vi "test Deploy Scripted System Definition.vi"(8 "error in (no error)":errorcluster, 11 "TestCase in":refnum<class "Switch Scripting System Tests.lvclass">=refnum) -> (0 "error out":errorcluster, 3 "TestCase out":refnum<class "Switch Scripting System Tests.lvclass">)   [LabVIEW 2017, in "Switch Scripting.lvlib" / "Switch Scripting System Tests.lvclass"]
uses:
  Switch Scripting System Tests.lvclass
  Switch Scripting System Tests.lvclass/Switch Scripting System Tests.ctl
  NationalInstruments.VeriStand.SystemDefinitionAPI
  <vilib>/addons/_JKI Toolkits/VI Tester/TestCase.llb/TestCase.lvclass
  C:/Program Files (x86)/National Instruments/LabVIEW 2017/vi.lib/addons/_JKI Toolkits/VI Tester/TestCase.llb/TestCase.lvclass
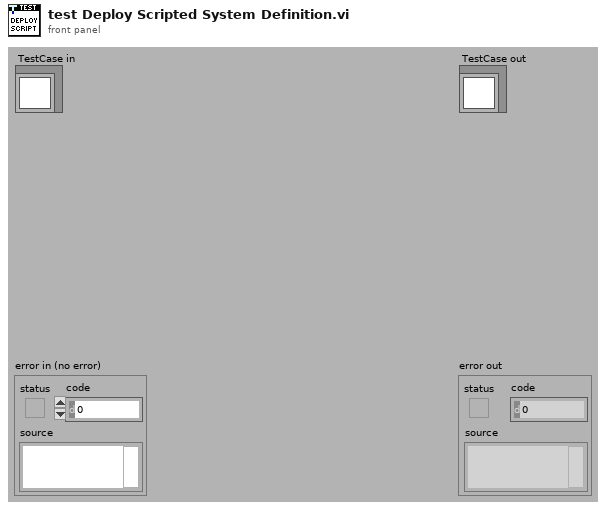
[diagram p1: front panel]
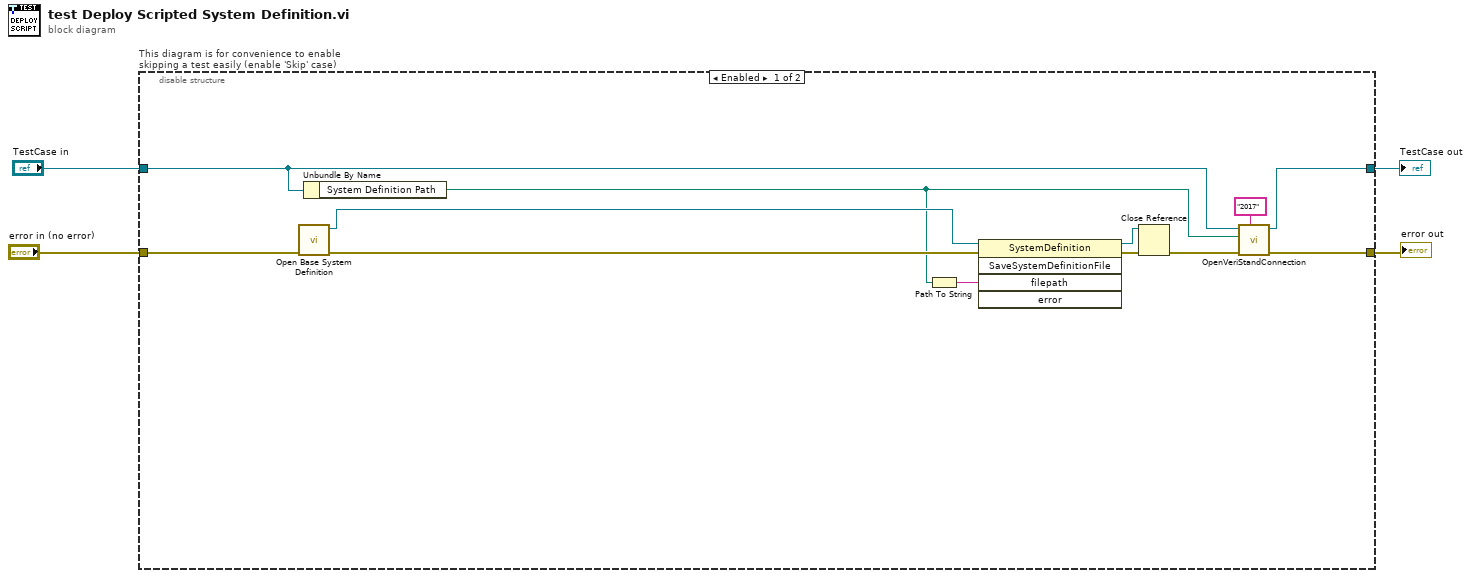
[diagram p0: block diagram]
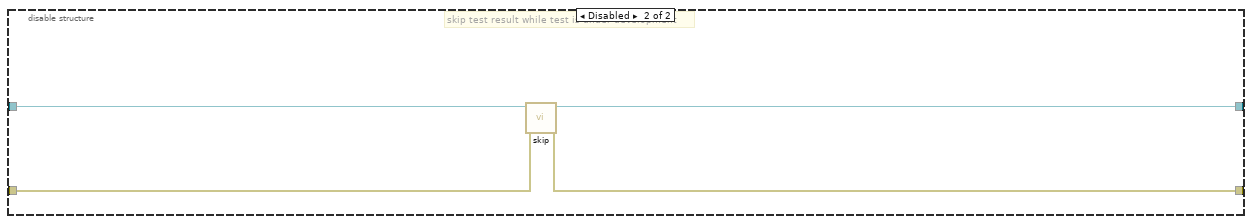
[diagram p2: hidden frame]
diagram:
  n1 = disable-structure "This diagram is for convenience to enable skipping a test easily (enable 'Skip' case)" shown="Enabled" {
    disable-tunnel: "TestCase in" -> [w14 w20]
    disable-tunnel: [w16 w18] -> w1
    disable-tunnel: [w15 w19] -> w3
    disable-tunnel: "error in (no error)" -> [w13 w17]
    frame Enabled {
      n2 = call "Open Base System Definition.vi"("error in (no error)"=w13) -> ("error out"=w12:errorcluster, "SystemDefinition"=w11:refnum<k24>)  [unwired: 8 in, 1 out]
      n3 = Unbundle By Name(w14) -> ("System Definition Path"=w7:path)
      n4 = Path To String(path=w7) -> (string=w8:string)
      n5 = invoke class="SystemDefinition" method="SaveSystemDefinitionFile"(reference=w11, error in=w12, "filepath"=w8) -> (reference out=w9:refnum<k24>, error out=w10:errorcluster)  [unwired: 2 in, 3 out]
      n6 = Close Reference(reference=w9, error in (no error)=w10) -> (error out=w5:errorcluster)
      n7 = call-dynamic "OpenVeriStandConnection.vi"("Minimum VeriStand Version (2015)"="2017", "error in (no error)"=w5, "System Definition File"=w7, "VeriStand Test Case in"=w14) -> ("error out"=w15:errorcluster, "VeriStand Test Case out"=w16:refnum<class "Switch Scripting System Tests.lvclass">)  [unwired: 5 in, 1 out]
    }
    frame Disabled {
      # "skip test result while test is under development"
      n8 = call <vilib>:"skip.vi"("error in (no error)"=w17, "TestCase in"=w20) -> ("error out"=w19:errorcluster, "TestCase out"=w18:refnum<class "Switch Scripting System Tests.lvclass">)  [unwired: 8 in]
    }
  }
  "error out" <- w3
  "TestCase out" <- w1
